vi "Begin.vi"() -> (0 "error out":errorcluster)   [LabVIEW 2011]
doc: "Called before other user functions, this VI is expected to open initial I/O refnums, load in file data, and do all program initialization. Notice that the <B>error out</B> terminal is simply used for data flow. Wiring it to other structures or subVIs ensures that this VI runs first."
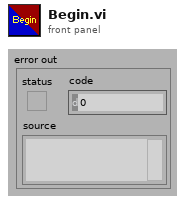
[diagram p1: front panel]
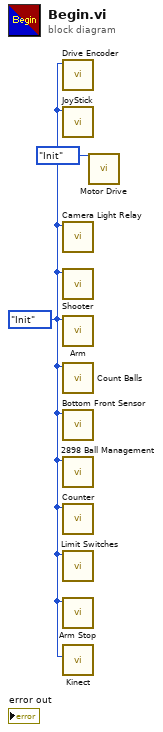
[diagram p0: block diagram]
diagram:
  w2 = enum16{"Init", "Run", "End"}."Init" ("Enum")
  n1 = call "Drive Encoder.vi"("Enum"=w2) -> ()  [unwired: 10 in, 1 out]
  n2 = call "JoyStick.vi"("Enum"=w2) -> ()  [unwired: 7 in, 4 out]
  n3 = call "Camera Light Relay.vi"("Enum"=w2) -> ()  [unwired: 11 in]
  n4 = call "Shooter.vi"("Enum"=w2) -> ()  [unwired: 10 in]
  n5 = call "Arm.vi"("Enum"=w2) -> ()  [unwired: 11 in]
  n6 = call "Count Balls.vi"("Mode"=w2) -> ()  [unwired: 8 in, 3 out]
  n7 = call "Bottom Front Sensor.vi"("Enum"=w2) -> ()  [unwired: 10 in, 1 out]
  n8 = call "2898 Ball Management.vi"("Enum"=w2) -> ()  [unwired: 11 in]
  n9 = call "Counter.vi"("Enum"=w2) -> ()  [unwired: 10 in, 1 out]
  n10 = call "Limit Switches.vi"("Enum"=w2) -> ()  [unwired: 9 in, 2 out]
  n11 = call "Arm Stop.vi"("Enum"=w2) -> ()  [unwired: 10 in]
  n12 = call "Kinect.vi"("Mode"=w2) -> ()  [unwired: 10 in, 1 out]
  n13 = call "Motor Drive.vi"("Enum"=enum16{"Init", "Run", "SetBrakeCoast", "End"}."Init") -> ()  [unwired: 11 in]
